vi "Puff_Dose_from_Continuous.vi"() -> (5 "Plug in titles":string[](array[string]), 7 "Plug in values":string[](array[string]))   [LabVIEW 2012]
uses:
  Globals/Meas_global.vi
  <vilib>/Analysis/baseanly.llb/Mean (DBL).vi
  <vilib>/Analysis/NI_AALBase.lvlib
panel:
  out "Dose per chop":dbl[](graph)
  out "Concentration Trace":dbl[](graph)
  in  "Chop length (s)":dbl
  out "fractional index or x":dbl
  out "D'/Dmean":dbl
  out "St Dev of Dose":dbl format="%0.2f"
  out "Mean Dose":dbl format="%0.2f"
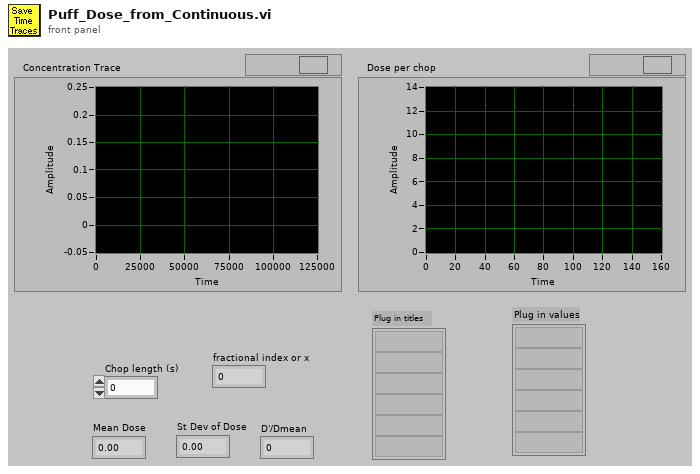
[diagram p1: front panel]
types:
  T1 = typedef "Time_Trace_Cluster.ctl" = cluster{"Weighting":dbl[], "Time (s)":dbl[], "Voltage":dbl[], "Eng Values":dbl[]}
  T2 = typedef "Analysis_info_cluster.ctl" = cluster{"Colour":u32, "Inst type":T3, "Inst name":string, "Symbol":string, "Code name":string, "Extra Info":string, "Inst Array":T4, "Extra Titles":string[], "Extra Values":string[], "U":dbl, "u^2":dbl, "u^3":dbl, "u^4":dbl, "Skew_u":dbl, "Kurt_u":dbl, "Sd Error in Mean":dbl, "% u'/U":dbl, "X":dbl, "Y":dbl, "Z":dbl, "Timescale integral to 25%":dbl, "Sd Error in Variance":dbl, "Calib File":path, "Calib Constants":dbl[], "Output Position":bool, "Full Stats":bool, "Av Sampling Rate":dbl, "Av No of Samples":dbl, "Total Meas Time (s)":dbl, "ADAM Ch Name":string}
  T3 = typedef "Inst_type.ctl" = enum16{"Propeller anemometer", "Raw voltage", "Pressure Transducer", "Pitot-static tube", "Preston tube", "Hot wire", "Cross wire 1", "Cross wire 2", "Generic Linear", "Generic Polynomial", "Generic BackPoly", "Fast FID", "Thermocouple", "Cold wire", "Pulsed Wire", "LDA Vel", "LDA Tran time", "LDA Arr time"}
  T4 = typedef "Instrument_Array.ctl" = enum16{"PWA", "LDA", "Analogue"}
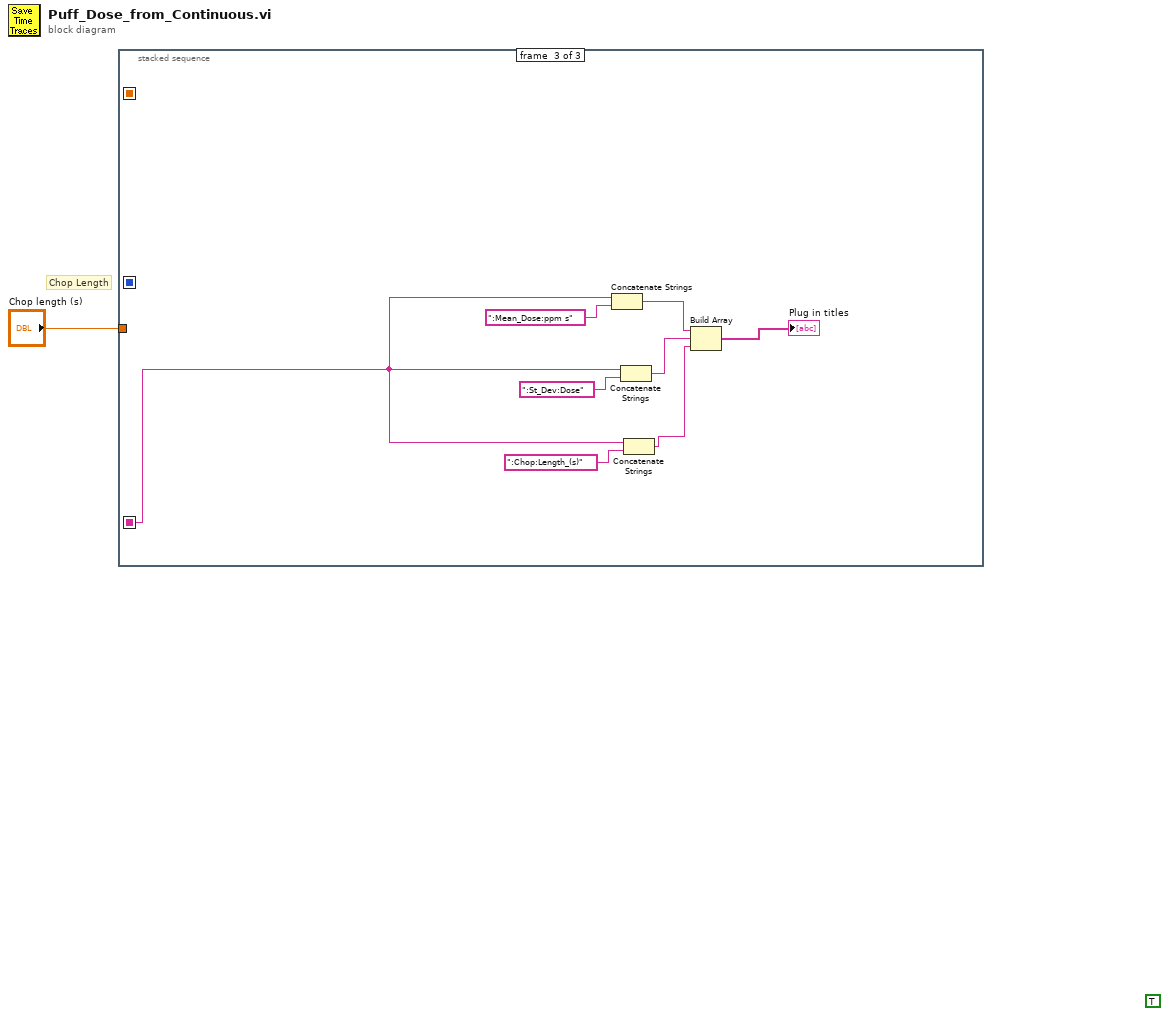
[diagram p0: block diagram]
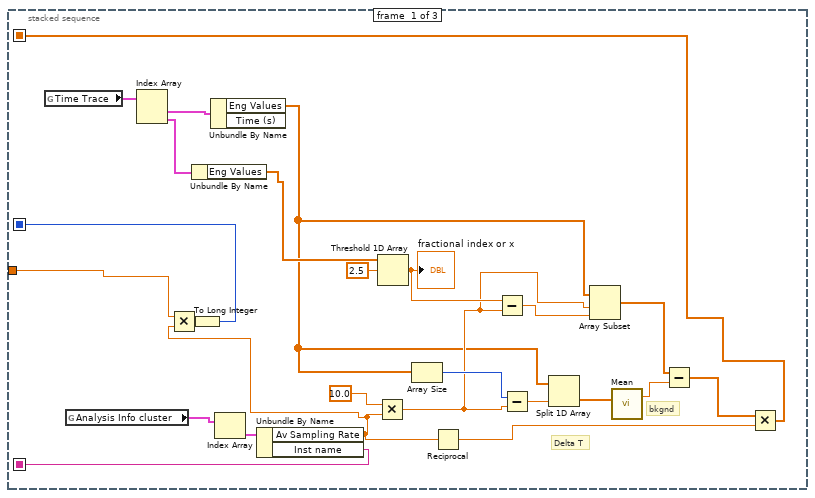
[diagram p2: hidden frame]
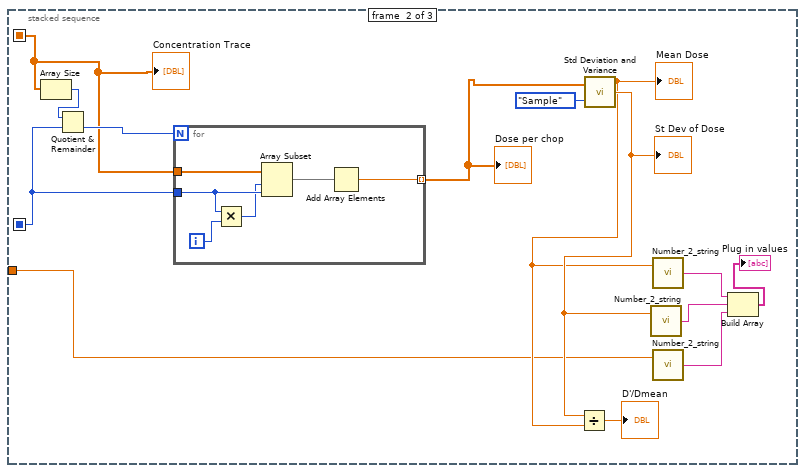
[diagram p3: hidden frame]
diagram:
  (unwired) TRUE
  # "Chop Length"
  n1 = stacked-sequence {
    seq-local: [w8 _ _] -> [_ _ w48]
    seq-local: [w6 _ _] -> [_ w27 _]
    seq-local: [w3 _ _] -> [_ w38 _]
    tunnel: "Chop length (s)" -> [w2 w30 _]
    frame #0 {
      # "bkgnd"
      # "Delta T"
      n2 = global read "Meas_global.vi" "Time Trace"() -> (w26:T1[])
      n3 = global read "Meas_global.vi" "Analysis Info cluster"() -> (w24:T2[])
      n4 = Index Array(array=w26) -> (element #1=w25:T1, element #2=w16:T1)  [unwired: 2 in]
      n5 = Unbundle By Name(w16) -> ("Eng Values"=w14:dbl[])
      n6 = Unbundle By Name(w25) -> ("Eng Values"=w10:dbl[])  [unwired: 1 out]
      n7 = Index Array(array=w24) -> (element=w23:T2)  [unwired: 1 in]
      n8 = Unbundle By Name(w23) -> ("Av Sampling Rate"=w5:dbl, "Inst name"=w8:string)
      n9 = Multiply(x=w2, y=w5) -> (x*y=w4:dbl)
      n10 = To Long Integer(number=w4) -> (32bit integer=w3:i32)
      n11 = Multiply(x=10.0, y=w5) -> (x*y=w11:dbl)
      n12 = Threshold 1D Array(2:2.5 ("threshold y"), 3:w14) -> (0:w13:dbl)  [unwired: 1 in]
      "fractional index or x" <- w13
      n13 = Array Size(array=w10) -> (size(s)=w21:i32)
      n14 = Reciprocal(x=w5) -> (1/x=w17:dbl)
      n15 = Subtract(x=w13, y=w11) -> (x-y=w12:dbl)
      n16 = Subtract(x=w21, y=w11) -> (x-y=w20:dbl)
      n17 = Split 1D Array(array=w10, index=w20) -> (second subarray=w19:dbl[])  [unwired: 1 out]
      n18 = Array Subset(array=w10, index=w11, length=w12) -> (w9:dbl[])
      n19 = call-poly <vilib>:"Mean.vi"("X"=w19) -> ("mean"=w18:dbl)  [unwired: 1 out]
      n20 = Subtract(x=w9, y=w18) -> (x-y=w7:dbl[])
      n21 = Multiply(x=w7, y=w17) -> (x*y=w6:dbl[])
    }
    frame #1 {
      n22 = Array Size(array=w27) -> (size(s)=w40:i32)
      n23 = Quotient & Remainder(x=w40, y=w38) -> (floor(x/y)=w39:i32)  [unwired: 1 out]
      n24 = for {
        N: w39 -> [_]
        tunnel: w27 -> [w46]
        tunnel: w38 -> [w44]
        tunnel: [w41] -> w28 mode=indexing
        i -> [w45]
        n25 = Multiply(x=w44, y=w45) -> (x*y=w43:i32)
        n26 = Array Subset(array=w46, index=w43, length=w44) -> (w42:dbl[])
        n27 = Add Array Elements(numeric array=w42) -> (sum=w41:dbl)
      }
      "Dose per chop" <- w28
      n28 = call <vilib>:"Std Deviation and Variance.vi"("X"=w28, "Weighting (Sample)"=enum16{"Sample", "Population"}."Sample") -> ("mean"=w35:dbl, "standard deviation"=w36:dbl)  [unwired: 1 out]
      "Mean Dose" <- w35
      "St Dev of Dose" <- w36
      n29 = Divide(x=w36, y=w35) -> (x/y=→"D'/Dmean":dbl)
      n30 = call "Number_2_string.vi"("number"=w36) -> ("String"=w32:string)  [unwired: 1 in]
      n31 = call "Number_2_string.vi"("number"=w35) -> ("String"=w33:string)  [unwired: 1 in]
      n32 = call "Number_2_string.vi"("number"=w30) -> ("String"=w29:string)  [unwired: 1 in]
      n33 = Build Array(w33, w32, w29) -> (→"Plug in values":string[])
      "Concentration Trace" <- w27
    }
    frame #2 {
      n34 = Concatenate Strings(w48, ":Mean_Dose:ppm s" ("string")) -> (w52:string)
      n35 = Concatenate Strings(w48, ":St_Dev:Dose" ("string")) -> (w53:string)
      n36 = Concatenate Strings(w48, ":Chop:Length_(s)" ("string")) -> (w47:string)
      n37 = Build Array(w52, w53, w47) -> (→"Plug in titles":string[])
    }
  }
